vi "Output Protection Status.vi"(8 "error in (no error)":errorcluster, 11 "VISA resource name":refnum<visa-resource-name>) -> (0 "error out":errorcluster, 1 "OCP Tripped?":bool, 2 "OVP Tripped?":bool, 3 "VISA resource name out":refnum<visa-resource-name>, 4 "OTP Tripped?":bool)   [LabVIEW 2014, in "Agilent N87XX Series.lvlib"]
doc: "Checks the status of the output protection and indicates if over voltage, current, or temperature have disabled the instrument. If none are tripped, the instrument is functioning normally. The Reset Output Protection VI will clear the output protection status."
uses:
  Agilent N87XX Series.lvlib
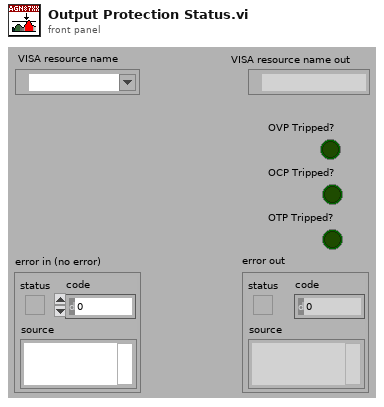
[diagram p1: front panel]
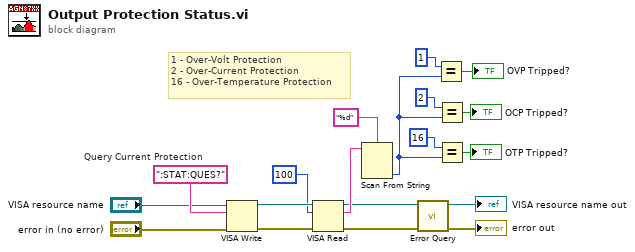
[diagram p0: block diagram]
diagram:
  w17 = ":STAT:QUES?"  # Query Current Protection
  # "1 - Over-Volt Protection\n2 - Over-Current Protection\n16 - Over-Temperature Protection"
  n1 = VISA Write(VISA resource name="VISA resource name", write buffer=w17, error in (no error)="error in (no error)") -> (VISA resource name out=w15:refnum<visa-resource-name>, error out=w16:errorcluster)  [unwired: 1 out]
  n2 = VISA Read(VISA resource name=w15, byte count=u32 100, error in (no error)=w16) -> (VISA resource name out=w1:refnum<visa-resource-name>, read buffer=w11:string, error out=w2:errorcluster)  [unwired: 1 out]
  n3 = Scan From String(format string="%d", input string=w11) -> (output 1=w3:i32)  [unwired: 3 in, 3 out]
  n4 = call "Error Query.vi"("error in (no error)"=w2, "VISA resource name"=w1) -> ("error out"=→"error out":errorcluster, "VISA resource name out"=→"VISA resource name out":refnum<visa-resource-name>)  [unwired: 6 in, 2 out]
  n5 = Equal?(x=1, y=w3) -> (x = y?=→"OVP Tripped?":bool)
  n6 = Equal?(x=2, y=w3) -> (x = y?=→"OCP Tripped?":bool)
  n7 = Equal?(x=16, y=w3) -> (x = y?=→"OTP Tripped?":bool)
